vi "DDE Request.vi"(7 "timeout (-1)":i32, 8 "error in (no error)":errorcluster, 10 "item":string, 11 "conversation refnum in":u32) -> (0 "error out":errorcluster, 2 "data":string, 3 "conversation refnum out":u32)   [LabVIEW 2018]
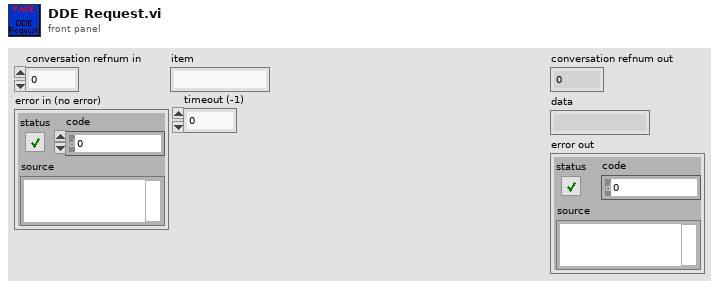
[diagram p1: front panel]
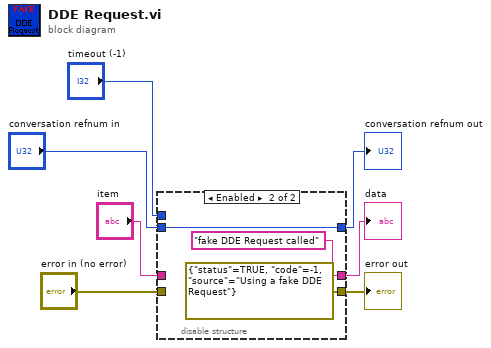
[diagram p0: block diagram]
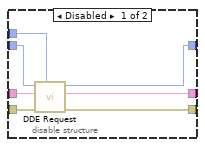
[diagram p2: hidden frame]
diagram:
  n1 = disable-structure shown="Enabled" {
    disable-tunnel: "conversation refnum in" -> [w14 w15]
    disable-tunnel: "error in (no error)" -> [w13 _]
    disable-tunnel: "item" -> [w12 _]
    disable-tunnel: "timeout (-1)" -> [w11 _]
    disable-tunnel: [w10 w15] -> w3
    disable-tunnel: [w9 "fake DDE Request called" ("source")] -> w2
    disable-tunnel: [w8 errorcluster {"status"=TRUE, "code"=-1, "source"="Using a fake DDE Request"} ("error out")] -> w1
    frame Disabled {
      n2 = call "DDE Request.vi"("timeout (-1)"=w11, "error in (no error)"=w13, "item"=w12, "conversation refnum in"=w14) -> ("error out"=w8:errorcluster, "data"=w9:string, "conversation refnum out"=w10:u32)  [unwired: 3 in]
    }
    frame Enabled {
    }
  }
  "conversation refnum out" <- w3
  "data" <- w2
  "error out" <- w1
